vi "Choreo_Choreo_AvailableTrajectories.vi"(8 "error in (no error)":errorcluster) -> (0 "error out":errorcluster, 3 "filenames":string[](array[string]), 4 "Path Out":path)   [LabVIEW 2019, in "ChoreoLib.lvlib"]
doc: "Fetches the names of all available trajectories in the deploy directory. \n\nInputs:\n - ErrorIn - cluster - standard error cluster. Can be used to force execution order.\n\nOutputs:\n - Filenames - string array - List of *.traj files found.\n - PathOut - path - the path that was searched.\n - ErrorOut - cluster - standard error cluster. Can be used to force execution order and check for errors."
uses:
  ChoreoLib.lvlib
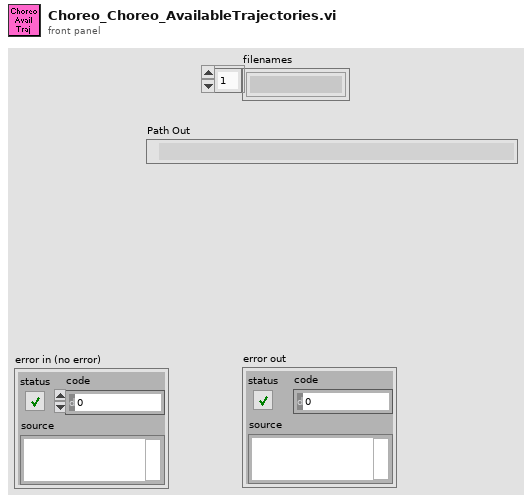
[diagram p1: front panel]
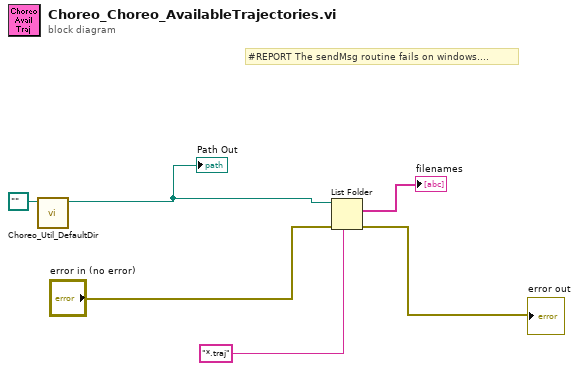
[diagram p0: block diagram]
diagram:
  # "#REPORT The sendMsg routine fails on windows...."
  n1 = call "Choreo_Util_DefaultDir.vi"("Path in"=path "") -> ("Path Out"=w5:path)  [unwired: 10 in]
  "Path Out" <- w5
  n2 = List Folder(path=w5, pattern="*.traj", error in="error in (no error)") -> (filenames=→"filenames":string[], error out=→"error out":errorcluster)  [unwired: 1 in, 2 out]
